vi "SWERVE_DRIVE_GET_SPEED_DEMAND.vi"() -> (0 "Drv Rotation Orentation Dmd":dbl, 1 "Drv Angular Vel Dmd":dbl, 2 "Drv Y Vel Dmd":dbl, 3 "Drv X Vel Dmd":dbl, 4 "Orientation Ctrl Enabled":bool)   [LabVIEW 2023]
uses:
  SWERVE_DRIVE_GLOBALS.vi
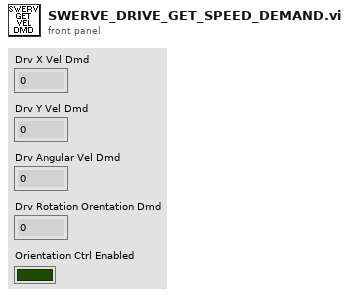
[diagram p1: front panel]
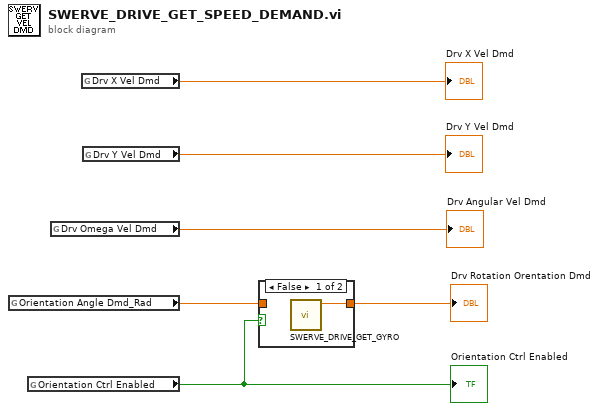
[diagram p0: block diagram]
diagram:
  n1 = global read "SWERVE_DRIVE_GLOBALS.vi" "Orientation Angle Dmd_Rad"() -> (w3:dbl)
  n2 = global read "SWERVE_DRIVE_GLOBALS.vi" "Orientation Ctrl Enabled"() -> (w2:bool)
  "Orientation Ctrl Enabled" <- w2
  n3 = global read "SWERVE_DRIVE_GLOBALS.vi" "Drv Omega Vel Dmd"() -> (→"Drv Angular Vel Dmd":dbl)
  n4 = global read "SWERVE_DRIVE_GLOBALS.vi" "Drv X Vel Dmd"() -> (→"Drv X Vel Dmd":dbl)
  n5 = global read "SWERVE_DRIVE_GLOBALS.vi" "Drv Y Vel Dmd"() -> (→"Drv Y Vel Dmd":dbl)
  n6 = case shown="False" w2 {
    tunnel: w3 -> [_ w8]
    tunnel: [w7 w8] -> w1
    frame False {
      n7 = call "SWERVE_DRIVE_GET_GYRO.vi"() -> ("Gyro Heading Radians"=w7:dbl)  [unwired: 11 in]
    }
    frame True {
    }
  }
  "Drv Rotation Orentation Dmd" <- w1
